vi "SendGetRequest.vi"(5 "path":string="contents", 6 "error in":errorcluster, 8 "repo":string="LabVIEWforRasPi", 9 "owner":string="labviewforRaspi") -> (0 "error out":errorcluster, 3 "url":string, 4 "body":string)   [LabVIEW 2014, in "GitHub API.lvlib"]
uses:
  GitHub API.lvlib
  <vilib>/httpClient/LabVIEWHTTPClient.lvlib
panel:
  # "https://api.github.com/repos/labviewforRaspi/LabVIEWforRasPi/contents/runtime/pyVI_1_0_0_755.tbz"
  # "https://api.github.com/repos/labviewforRaspi/LabVIEWforRasPi/contents"
  # "https://api.github.com/repos/labviewforRaspi/LabVIEWforRasPi/git/trees/1ae79e1da9e53f466e72627d3951b054781a98b9"
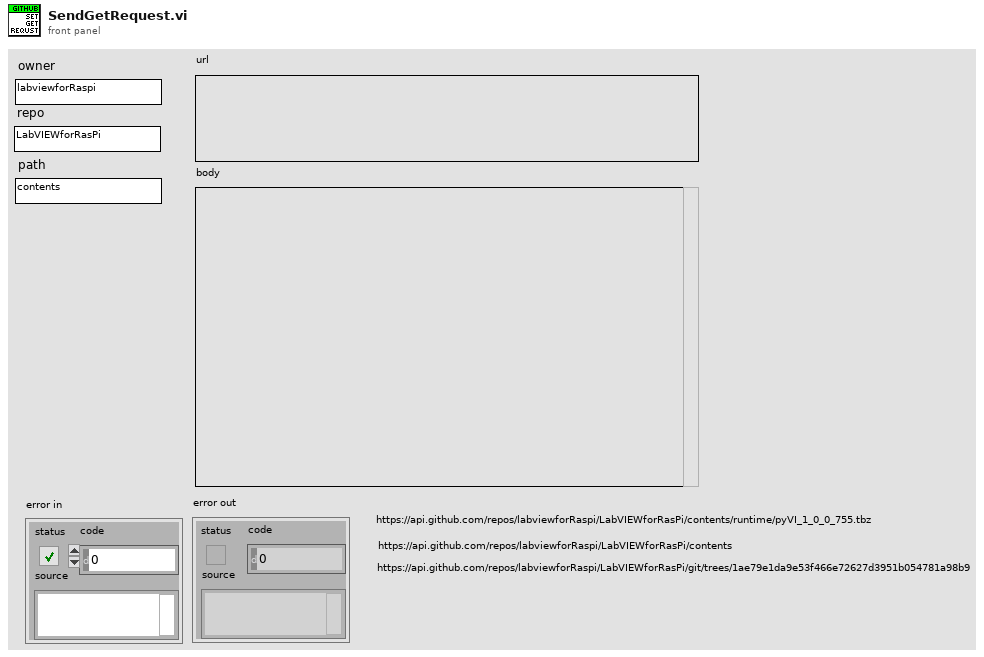
[diagram p1: front panel]
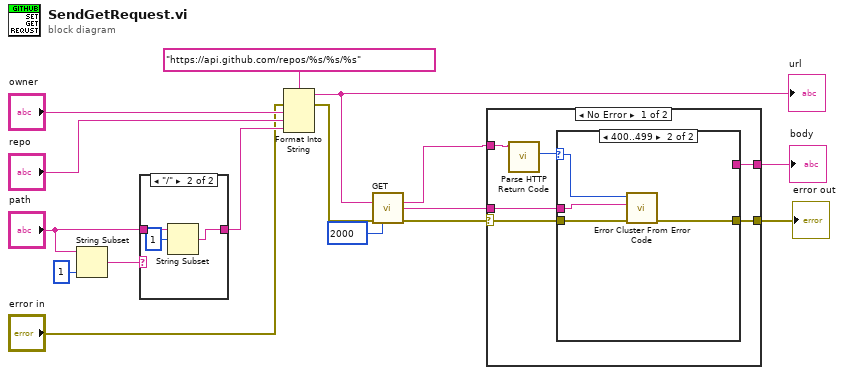
[diagram p0: block diagram]
diagram:
  n1 = String Subset(string="path", length (rest)=1 ("length (rest)")) -> (substring=w13:string)  [unwired: 1 in]
  n2 = case shown="\"/\"" w13 {
    tunnel: "path" -> [w17 w20]
    tunnel: [w17 w19] -> w11
    frame Default {
    }
    frame "/" {
      n3 = String Subset(string=w20, offset (0)=1) -> (substring=w19:string)  [unwired: 1 in]
    }
  }
  n4 = Format Into String(format string="https://api.github.com/repos/%s/%s/%s", error in="error in", "owner", "repo", w11) -> (resulting string=w9:string, error out=w8:errorcluster)  [unwired: 1 in]
  "url" <- w9
  n5 = call <vilib>:"GET.vi"("url"=w9, "error in (no error)"=w8, "timeout (10000)"=2000) -> ("headers"=w1:string, "body"=w6:string, "error out"=w5:errorcluster)  [unwired: 9 in, 1 out]
  n6 = case shown="No Error" w5 {
    selector: w5 -> [w26 w33]
    tunnel: w6 -> [w25 _]
    tunnel: [w24 w33] -> w3
    tunnel: [w23 _] -> w4
    tunnel: w1 -> [w22 _]
    frame No Error {
      n7 = call "Parse HTTP Return Code.vi"("headers"=w22) -> ("code"=w21:i32)  [unwired: 8 in, 2 out]
      n8 = case shown="400..499" w21 {
        selector: w21 -> [_ w32]
        tunnel: w26 -> [w27 w31]
        tunnel: w25 -> [w28 w30]
        tunnel: [w27 w29] -> w24
        tunnel: [w28 _] -> w23
        frame Default {
        }
        frame 400..499 {
          n9 = call <vilib>:"Error Cluster From Error Code.vi"("error in (no error)"=w31, "error message (\"\")"=w30, "error code (0)"=w32) -> ("error out"=w29:errorcluster)  [unwired: 6 in]
        }
      }
    }
    frame Error {
    }
  }
  "body" <- w4
  "error out" <- w3
